vi "de_turboCode.vi"(8 "error in":errorcluster, 10 "poutput":dbl[](array[numeric]), 11 "Path In":path) -> (0 "error out":errorcluster, 2 "decodedBit":dbl[](array[numeric]), 3 "Path Out":path)   [LabVIEW 2015]
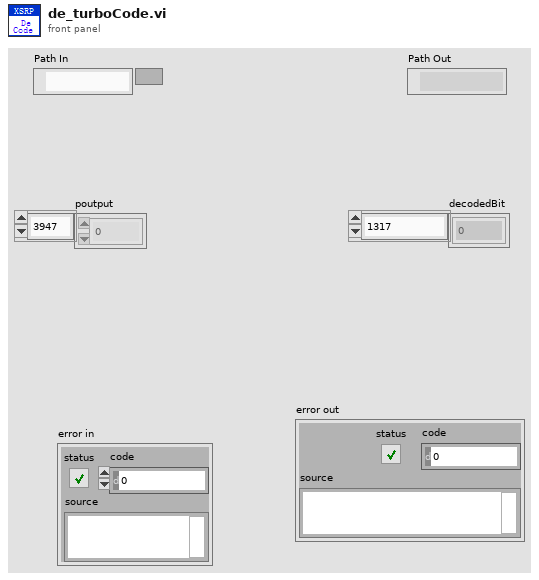
[diagram p1: front panel]
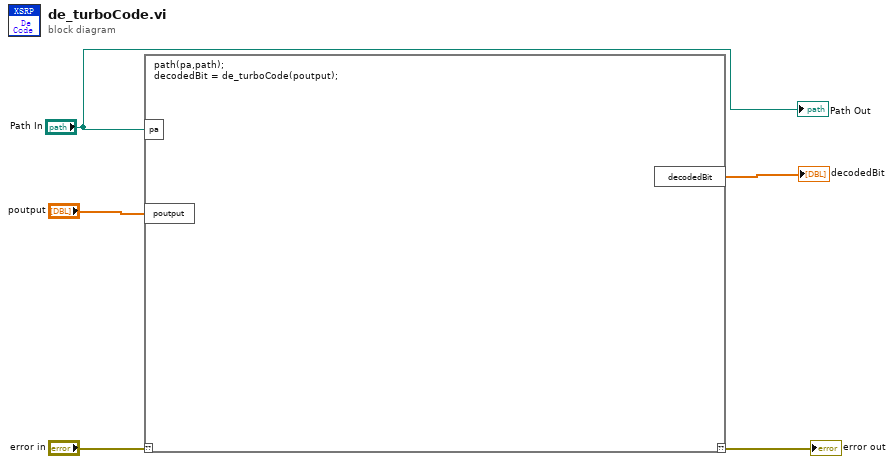
[diagram p0: block diagram]
diagram:
  n1 = script code="path(pa,path);\ndecodedBit = de_turboCode(poutput);"("??"="error in", "pa"="Path In", "poutput"="poutput") -> ("??"=→"error out":errorcluster, "decodedBit"=→"decodedBit":dbl[])
  "Path Out" <- "Path In"
